vi "Troubleshoot 2.vi"(8 "error in (no error)":errorcluster, 10 "Targets in":T1 {"Filtered Targets"."IP Mode" items=["Static"=1, "DHCP/Link-Local"=2, "Link-Local Only"=4, "DHCP Only"=8]}, 11 "Ctl Refs in":T6) -> (0 "error out":errorcluster, 1 "User State":T4, 2 "Targets out":T1 {"Filtered Targets"."IP Mode" items=["Static"=1, "DHCP/Link-Local"=2, "Link-Local Only"=4, "DHCP Only"=8]}, 3 "Ctl Refs out":T6, 4 "Execution State":T5)   [LabVIEW 2013]
uses:
  Controls/Refs.ctl
  Controls/Button Refs.ctl
  Controls/Tab Ctl Refs.ctl
  types/TabStateType.ctl
  Controls/Indicator Refs.ctl
  Controls/Slider Refs.ctl
  Controls/Control Refs.ctl
  Controls/Targets.ctl
  Controls/Detected.ctl
  types/MAX Sys Cfg Target Information.ctl
  types/ExecutionStateType.ctl
  types/UserStateType.ctl
panel:
  in  "stop_loop":bool
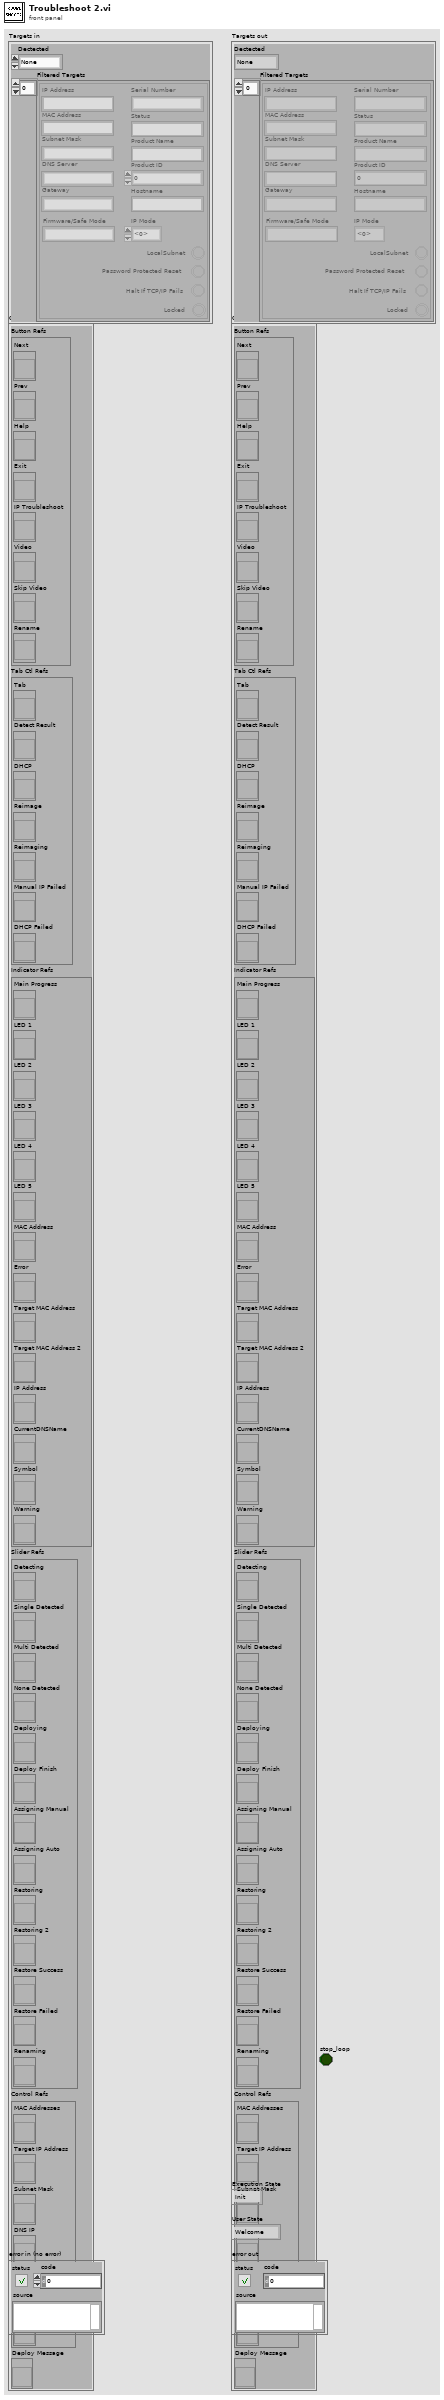
[diagram p1: front panel]
types:
  T1 = typedef "Targets.ctl" = cluster{"Dectected":T2, "Filtered Targets":T3[]}
  T2 = typedef "Detected.ctl" = enum16{"None", "Failed", "Single", "Multi"}
  T3 = typedef "MAX Sys Cfg Target Information.ctl" = cluster{"MAC Address":string, "IP Address":string, "Status":string, "Product Name":string, "Hostname":string, "Firmware/Safe Mode":string, "Subnet Mask":string, "Gateway":string, "DNS Server":string, "Serial Number":string, "Product ID":u32, "Locked ":bool, "LocalSubnet":bool, "Halt If TCP/IP Fails":bool, "Password Protected Reset":bool, "IP Mode":i32}
  T4 = typedef "UserStateType.ctl" = enum16{"Welcome", "Instructions", "Detect", "Deploy", "Success"}
  T5 = typedef "ExecutionStateType.ctl" = enum16{"Init", "Welcome", "Idle", "Detect", "Run Detection", "Detect Fail", "Detect One", "Detect Mult", "Deploy", "DHCP", "Static IP", "Run Deployment", "Connect Verify", "Exit", "Video Wait", "Success", "Troubleshoot", "Troubleshoot 2", "RenameDNS"}
  T6 = typedef "Refs.ctl" = cluster{"Button Refs":T7, "Tab Ctl Refs":T8, "Indicator Refs":T9, "Slider Refs":T10, "Control Refs":T11, "Deploy Message":refnum<vi>}
  T7 = typedef "Button Refs.ctl" = cluster{"Next":refnum<vi>, "Prev":refnum<vi>, "Help":refnum<vi>, "Exit":refnum<vi>, "IP Troubleshoot":refnum<vi>, "Video":refnum<vi>, "Skip Video":refnum<vi>, "Rename":refnum<vi>}
  T8 = typedef "Tab Ctl Refs.ctl" = cluster{"Tab":refnum<vi>, "Detect Result":refnum<vi>, "DHCP":refnum<vi>, "Reimage":refnum<vi>, "Reimaging":refnum<vi>, "Manual IP Failed":refnum<vi>, "DHCP Failed":refnum<vi>}
  T9 = typedef "Indicator Refs.ctl" = cluster{"Main Progress":refnum<vi>, "LED 1":refnum<vi>, "LED 2":refnum<vi>, "LED 3":refnum<vi>, "LED 4":refnum<vi>, "LED 5":refnum<vi>, "MAC Address":refnum<vi>, "Error":refnum<vi>, "Target MAC Address":refnum<vi>, "Target MAC Address 2":refnum<vi>, "IP Address":refnum<vi>, "CurrentDNSName":refnum<vi>, "Symbol":refnum<vi>, "Warning":refnum<vi>}
  T10 = typedef "Slider Refs.ctl" = cluster{"Detecting":refnum<vi>, "Single Detected":refnum<vi>, "Multi Detected":refnum<vi>, "None Detected":refnum<vi>, "Deploying":refnum<vi>, "Deploy Finish":refnum<vi>, "Assigning Manual":refnum<vi>, "Assigning Auto":refnum<vi>, "Restoring":refnum<vi>, "Restoring 2":refnum<vi>, "Restore Success":refnum<vi>, "Restore Failed":refnum<vi>, "Renaming":refnum<vi>}
  T11 = typedef "Control Refs.ctl" = cluster{"MAC Addresses":refnum<vi>, "Target IP Address":refnum<vi>, "Subnet Mask":refnum<vi>, "DNS IP":refnum<vi>, "Default Gateway":refnum<vi>, "DNSName":refnum<vi>}
  T12 = enum32{"Welcome", "Instructions", "Detect", "Run Detection", "Detect Result", "Deploy", "Run Deployment", "Connect Verify", "Success", "DHCP", "Troubleshoot", "System Restore"}
  T13 = enum32{"Welcome", "Instructions", "Detect", "Run Detection", "Detect Result", "Deploy", "Run Deployment", "Connect Verify", "Success", "DHCP", "Troubleshoot", "System Restore", "Error", "Video"}
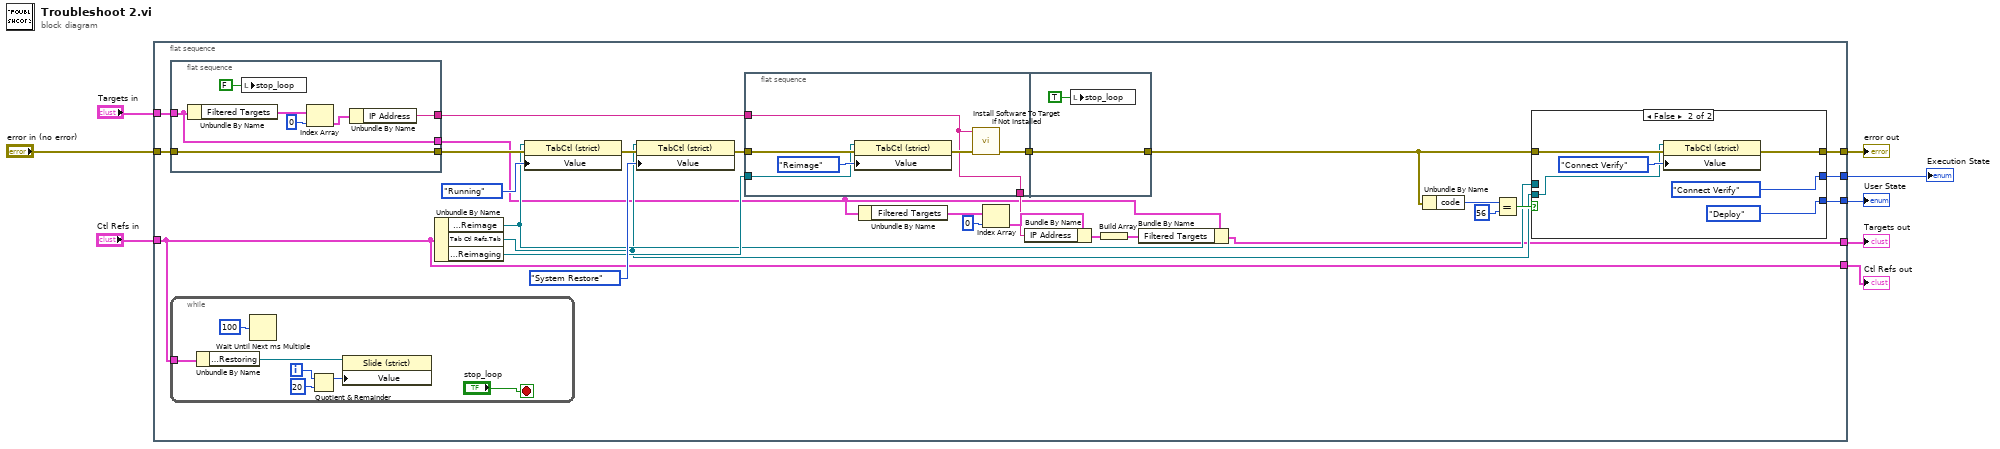
[diagram p0: block diagram]
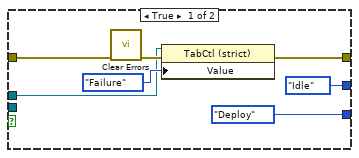
[diagram p2: hidden frame]
diagram:
  n1 = flat-sequence {
    tunnel: "Targets in" -> [w36]
    tunnel: "error in (no error)" -> [w35]
    tunnel: [w34] -> w3
    tunnel: [w20] -> w4
    tunnel: [w19] -> w5
    tunnel: [w11] -> w6
    tunnel: "Ctl Refs in" -> [w10]
    tunnel: [w10] -> w8
    frame #0 {
      n2 = flat-sequence {
        tunnel: w36 -> [w60]
        tunnel: [w60] -> w13
        tunnel: [w62] -> w33
        tunnel: w35 -> [w62]
        tunnel: [w61] -> w24
        frame #0 {
          n3 = Unbundle By Name(w60) -> ("Filtered Targets"=w59:T3[])
          n4 = local write "stop_loop"(FALSE ("stop_loop")) -> ()
          n5 = Index Array(array=w59, index=0) -> (element=w63:T3)
          n6 = Unbundle By Name(w63) -> ("IP Address"=w61:string)
        }
      }
      n7 = while {
        tunnel: w10 -> [w68]
        i -> [w69]
        stop <- "stop_loop" stop-if-true
        n8 = Unbundle By Name(w68) -> ("Slider Refs.Restoring"=w67:refnum<vi>)
        n9 = Wait Until Next ms Multiple(millisecond multiple=u32 100 ("milliseconds to wait")) -> ()  [unwired: 1 out]
        n10 = Quotient & Remainder(x=w69, y=20) -> (x-y*floor(x/y)=w66:i32)  [unwired: 1 out]
        n11 = property class="Slide (strict)"(reference=w67, "Value"=w66) -> ()  [unwired: 1 in, 2 out]
      }
      n12 = Unbundle By Name(w10) -> ("Tab Ctl Refs.Reimage"=w16:refnum<vi>, "Tab Ctl Refs.Tab"=w15:refnum<vi>, "Tab Ctl Refs.Reimaging"=w17:refnum<vi>)
      n13 = property on="Property Node" class="TabCtl (strict)"(reference=w16, error in=w33, "Value"=enum32{"Running", "Success", "Failure"}."Running" ("Reimage Tabs")) -> (error out=w23:errorcluster)  [unwired: 1 out]
      n14 = property on="Property Node" class="TabCtl (strict)"(reference=w15, error in=w23, "Value"=T12."System Restore" ("Tab Control")) -> (error out=w22:errorcluster)  [unwired: 1 out]
      n15 = flat-sequence {
        tunnel: [w53] -> w9
        tunnel: w22 -> [w54]
        tunnel: w24 -> [w50]
        tunnel: [w50] -> w18
        tunnel: w17 -> [w51]
        tunnel: [w57] -> w28
        tunnel: w9 -> [w57]
        frame #0 {
          n16 = property on="Property Node" class="TabCtl (strict)"(reference=w51, error in=w54, "Value"=enum32{"Reformat", "Reimage", "IP Config"}."Reimage" ("Reimaging Tabs")) -> (error out=w52:errorcluster)  [unwired: 1 out]
          n17 = call "Install Software To Target if Not Installed.vi"("error in (no error)"=w52, "MAC Address"=w50) -> ("error out"=w53:errorcluster)  [unwired: 8 in, 1 out]
        }
        frame #1 {
          n18 = local write "stop_loop"(TRUE ("stop_loop")) -> ()
        }
      }
      n19 = Unbundle By Name(w13) -> ("Filtered Targets"=w14:T3[])
      n20 = Index Array(array=w14, index=0) -> (element=w26:T3)
      n21 = Bundle By Name(cluster=w26, "IP Address"=w18) -> (w25:T3)
      n22 = Build Array(w25) -> (w12:T3[])
      n23 = Bundle By Name(cluster=w13, "Filtered Targets"=w12) -> (w11:T1)
      n24 = Unbundle By Name(w28) -> ("code"=w31:i32)
      n25 = Equal?(x=w31, y=56) -> (x = y?=w30:bool)
      n26 = case shown="False" w30 {
        tunnel: w28 -> [w41 w47]
        tunnel: [w42 w46] -> w34
        tunnel: [UserStateType."Deploy" ("Enum 2") UserStateType."Deploy" ("Enum 2")] -> w20
        tunnel: [ExecutionStateType."Idle" ("Enum") ExecutionStateType."Connect Verify" ("Enum")] -> w19
        tunnel: w16 -> [w37 _]
        tunnel: w15 -> [_ w44]
        frame True {
          n27 = call <vilib>:"Clear Errors.vi"("error in (no error)"=w41) -> ("error out"=w40:errorcluster)  [unwired: 6 out]
          n28 = property on="Property Node" class="TabCtl (strict)"(reference=w37, error in=w40, "Value"=enum32{"Running", "Success", "Failure"}."Failure" ("Reimage Tabs")) -> (error out=w42:errorcluster)  [unwired: 1 out]
        }
        frame False {
          n29 = property on="Property Node" class="TabCtl (strict)"(reference=w44, error in=w47, "Value"=T13."Connect Verify" ("Tab Control")) -> (error out=w46:errorcluster)  [unwired: 1 out]
        }
      }
    }
  }
  "Ctl Refs out" <- w8
  "Targets out" <- w6
  "Execution State" <- w5
  "User State" <- w4
  "error out" <- w3
